vi "UPRcontroller_v00_basedonlsmv66.vi"() -> ()   [LabVIEW 2015] (continued)
                                n2048 = call "2pparameters.vi"("Params in"=w5216, "command"="set") -> ()  [unwired: 1 out]
                                }
                                frame #1 {
                                n2049 = call "waveformparamsv2.vi"("command"="rem DO", "index"=w5227) -> ()  [unwired: 3 in, 3 out]
                                }
                                frame #2 {
                                n2050 = call "waveformsDObuffer.vi"("command"="get") -> ("DO wf out"=w5233:digitalwaveform[])  [unwired: 1 in]
                                n2051 = Delete From Array(array=w5233, length=1, index=w5232) -> (array with subset deleted=w5229:digitalwaveform[])  [unwired: 1 out]
                                n2052 = call "waveformsDObuffer.vi"("DO wf in"=w5229, "command"="set") -> ()  [unwired: 1 out]
                                }
                                }
                                }
                                frame 2 {
                                n2053 = stacked-sequence {
                                tunnel: w5236 -> [_ _ w5249]
                                tunnel: w5235 -> [_ w5247 _]
                                frame #0 {
                                n2054 = call "configuration.vi"("command"="get") -> ("config out"=w5238:T14)  [unwired: 2 in, 1 out]
                                n2055 = Unbundle By Name(w5238) -> ("LT timestamp"=w5237:u32)
                                n2056 = call "2pparameters.vi"("command"="get") -> ("params out"=w5242:T12)  [unwired: 1 in]
                                n2057 = in-place {
                                in-place-border: w5237 -> [w5246]
                                n2058 = in-place-cluster #42(w5242) -> ("aDO"=w5245:u32[])
                                n2059 = call "add channel to active arrayv2.vi"("line array in"=w5245, "line to add"=w5246) -> ("line array out"=w5244:u32[])  [unwired: 2 out]
                                n2060 = in-place-cluster #42("aDO"=w5244) -> (w5240:T12)
                                }
                                n2061 = call "2pparameters.vi"("Params in"=w5240, "command"="set") -> ()  [unwired: 1 out]
                                }
                                frame #1 {
                                n2062 = call "waveformparamsv2.vi"("command"="add DO", "add DO"=w5247) -> ()  [unwired: 3 in, 3 out]
                                }
                                frame #2 {
                                n2063 = call "waveformsDObuffer.vi"("command"="get") -> ("DO wf out"=w5252:digitalwaveform[])  [unwired: 1 in]
                                n2064 = Build Array (concatenate)(w5252, w5249) -> (w5251:digitalwaveform[])
                                n2065 = call "waveformsDObuffer.vi"("DO wf in"=w5251, "command"="set") -> ()  [unwired: 1 out]
                                }
                                }
                                }
                                frame 0 {
                                n2066 = stacked-sequence {
                                seq-local: [w5258 _ _] -> [_ w5268 w5285]
                                tunnel: w5257 -> [_ _ _]
                                tunnel: w5256 -> [_ _ _]
                                tunnel: w5255 -> [_ w5265 _]
                                tunnel: w5254 -> [_ _ w5284]
                                frame #0 {
                                n2067 = call "configuration.vi"("command"="get") -> ("config out"=w5263:T14)  [unwired: 2 in, 1 out]
                                n2068 = Unbundle By Name(w5263) -> ("LT timestamp"=w5259:u32)
                                n2069 = call "2pparameters.vi"("command"="get") -> ("params out"=w5262:T12)  [unwired: 1 in]
                                n2070 = Unbundle By Name(w5262) -> ("aDO"=w5260:u32[])
                                n2071 = Search 1D Array(1D array=w5260, element=w5259) -> (index of element=w5258:i32)  [unwired: 1 in]
                                }
                                frame #1 {
                                n2072 = local read "Measurement"() -> (w5267:T4)
                                n2073 = To Unsigned Long Integer(number=w5267) -> (unsigned 32bit integer=w5266:u32)
                                n2074 = case shown="5..7" w5266 {
                                tunnel: w5268 -> [_ w5272]
                                tunnel: w5265 -> [_ w5269]
                                frame 0..4, Default {
                                }
                                frame 5..7 {
                                n2075 = Index Array(array=w5269, index=0) -> (element=w5270:T21)
                                n2076 = call "waveformparamsv2.vi"("command"="get") -> ("Params out"=w5275:T17)  [unwired: 4 in, 2 out]
                                n2077 = in-place {
                                in-place-border: w5272 -> [w5279]
                                in-place-border: w5270 -> [w5277]
                                n2078 = in-place-cluster #43(w5275) -> ("DO parameters"=w5280:T20)
                                n2079 = in-place {
                                in-place-border: w5277 -> [w5281]
                                n2080 = in-place-array #44(w5280, w5279) -> ()  [unwired: 1 out]
                                n2081 = in-place-array #44(w5281) -> (w5278:T20)  [unwired: 1 out]
                                }
                                n2082 = in-place-cluster #43("DO parameters"=w5278) -> (w5273:T17)
                                }
                                n2083 = call "waveformparamsv2.vi"("command"="set", "Params in"=w5273) -> ()  [unwired: 3 in, 3 out]
                                }
                                }
                                }
                                frame #2 {
                                n2084 = local read "Measurement"() -> (w5283:T4)
                                n2085 = To Unsigned Long Integer(number=w5283) -> (unsigned 32bit integer=w5282:u32)
                                n2086 = case shown="5..7" w5282 {
                                tunnel: w5285 -> [_ w5289]
                                tunnel: w5284 -> [_ w5287]
                                frame 0..4, Default {
                                }
                                frame 5..7 {
                                n2087 = Index Array(array=w5287, index=0) -> (element=w5286:digitalwaveform)
                                n2088 = call "waveformsDObuffer.vi"("command"="get") -> ("DO wf out"=w5291:digitalwaveform[])  [unwired: 1 in]
                                n2089 = Replace Array Subset(array=w5291, new element=w5286, index=w5289) -> (w5293:digitalwaveform[])
                                n2090 = call "waveformsDObuffer.vi"("DO wf in"=w5293, "command"="set") -> ()  [unwired: 1 out]
                                }
                                }
                                }
                                }
                                }
                                }
                              }
                              frame #4 {
                                n2091 = call "Used AO lines.vi"() -> ("used AO names"=w5296:string[], "used AO lines"=w5294:tag[])  [unwired: 2 in]
                                n2092 = control-ref of="Analog Lines Plot"() -> (w5295:refnum<vi>)
                                n2093 = control-ref of="Digital Lines Plot"() -> (w5297:refnum<vi>)
                                n2094 = call "Used DO lines.vi"() -> ("used DO names"=w5298:string[], "used DO lines"=w5299:tag[])  [unwired: 2 in]
                                n2095 = local write "Analog Used Lines"(w5294) -> ()
                                n2096 = local write "Analog Used Names"(w5296) -> ()
                                n2097 = local write "Digital Used Lines"(w5299) -> ()
                                n2098 = local write "Digital Used Names"(w5298) -> ()
                                n2099 = call "prepDOWaveplot.vi"("DigitalGraph in"=w5297, "used DO names"=w5298) -> ()  [unwired: 1 in]
                                n2100 = call "prepAOWaveplot.vi"("WaveformGraph in"=w5295, "Analog Used Names"=w5296) -> ()  [unwired: 1 in]
                              }
                              frame #5 {
                                # "source of crashing?"
                                n2101 = local read "Meastab"() -> (w5314:enum32{"X-Y Image", "Linescan", "Timetrace"})
                                n2102 = property on="refwf" class="Ring (strict)"() -> ("RingText.Text"=w5311:string)  [unwired: 2 in, 2 out]
                                n2103 = case shown="\"Timetrace\"" w5314 {
                                tunnel: [w5316 w5317] -> w5315
                                frame "X-Y Image", Default {
                                n2104 = local read "Sampling rate"() -> (w5316:dbl)
                                }
                                frame "Timetrace" {
                                n2105 = local read "srateAODOtt"() -> (w5317:dbl)
                                }
                                }
                                n2106 = call "waveformsAObuffer.vi"("command"="get") -> ("AO wf out"=w5302:waveform(dbl)[])  [unwired: 1 in]
                                n2107 = local read "wavdet"() -> (w5312:bool)
                                n2108 = call "waveformsDObuffer.vi"("command"="get") -> ("DO wf out"=w5306:digitalwaveform[])  [unwired: 1 in]
                                n2109 = call "correctwaveformsizetemp.vi"("new sampling frequency (Hz)"=w5315, "start"=FALSE, "reference waveforms to"=w5311, "Analog waveforms in"=w5302, "stop"=TRUE, "Digital waveforms in"=w5306) -> ("analog wf out"=w5308:waveform(dbl)[], "Digital wf out"=w5310:digitalwaveform[], "measpoints"=w5313:i32)
                                n2110 = local write "Analog Lines Plot"(w5308) -> ()
                                n2111 = call "GetNumCamFramesv2.vi"("Digital Waveform Graph"=w5310) -> ("Numeric"=w5309:i32)  [unwired: 10 in]
                                n2112 = local write "Digital Lines Plot"(w5310) -> ()
                                n2113 = call "waveformsDObuffer.vi"("DO wf in"=w5310, "command"="set") -> ()  [unwired: 1 out]
                                n2114 = call "waveformsAObuffer.vi"("AO wf in"=w5308, "command"="set") -> ()  [unwired: 1 out]
                                n2115 = local write "Total Camera Frames"(w5309) -> ()
                                n2116 = case shown="True" w5312 {
                                tunnel: w5313 -> [_ w5318]
                                frame False {
                                }
                                frame True {
                                n2117 = local write "# of frames"(w5318) -> ()
                                }
                                }
                              }
                            }
                          }
                          frame #9 {
                            w5328 = FALSE ("Value (Signaling)")
                            # "Save parameters, reset system..."
                            n2118 = local read "save\ndata"() -> (w5323:bool)
                            n2119 = case shown="True" w5323 {
                              tunnel: w5322 -> [_ w5335]
                              frame False {
                              }
                              frame True {
                                n2120 = call "closebinaryfiles.vi"() -> ()  [unwired: 12 in]
                                n2121 = local read "filename prefix"() -> (w5336:string)
                                n2122 = local read "data dir"() -> (w5337:path)
                                n2123 = disable-structure shown="Disabled" {
                                disable-tunnel: w5336 -> [w5340 _]
                                disable-tunnel: w5337 -> [w5339 _]
                                disable-tunnel: w5335 -> [w5338 _]
                                frame Disabled {
                                n2124 = call "saveparams.vi"("timestamp"=w5338, "filename prefix in"=w5340, "data dir in"=w5339) -> ()  [unwired: 1 in]
                                }
                                frame Enabled {
                                }
                                }
                                n2125 = call "saveparams_andscanpattern.vi"("timestamp"=w5335, "filename prefix in"=w5336, "data dir in"=w5337) -> ()  [unwired: 1 in]
                              }
                            }
                            n2126 = call "2pparameters.vi"("command"="get") -> ("params out"=w5319:T12)  [unwired: 1 in]
                            n2127 = Unbundle By Name(w5319) -> ("auto OD"=w5320:bool)
                            n2128 = case shown="True" w5320 {
                              frame False {
                              }
                              frame True {
                                n2129 = call "configuration.vi"("command"="get") -> ("config out"=w5331:T14)  [unwired: 2 in, 1 out]
                                n2130 = call "2pparameters.vi"("command"="get") -> ("params out"=w5334:T12)  [unwired: 1 in]
                                n2131 = Unbundle By Name(w5331) -> ("contour OD"=w5329:u16)
                                n2132 = Unbundle By Name(w5334) -> ("ODfilt"=w5330:u16)
                                n2133 = call "filterwheelcontrol_nothorlabslib.vi"("Current OD filt"=w5329, "New ODfilt"=w5330) -> ()  [unwired: 1 in]
                              }
                            }
                            n2134 = property on="Start" class="Bool (strict)"("Val(Sgnl)"=w5328) -> ()  [unwired: 2 in, 2 out]
                            n2135 = property on="Start" class="Bool (strict)"("Visible"=TRUE, "DisabledEnum"=T8."Enabled" ("Disabled")) -> ()  [unwired: 2 in, 2 out]
                            n2136 = property on="Stop" class="Bool (strict)"("Val(Sgnl)"=w5328) -> ()  [unwired: 2 in, 2 out]
                            n2137 = property on="Stop" class="Bool (strict)"("Visible"=FALSE, "DisabledEnum"=T8."Disabled" ("Disabled")) -> ()  [unwired: 2 in, 2 out]
                          }
                          frame #10 {
                            w5343 = T24 2 items=["no dialog", "OK message", "continue or stop message", "OK message + warnings", "continue/stop + warnings"] ("type of dialog (OK msg:1)")
                            # "Error Handling"
                            n2138 = call "displayerrors.vi"() -> ("error IO"=w5344:errorcluster)
                            n2139 = call <vilib>:"General Error Handler.vi"("type of dialog (OK msg:1)"=w5343, "error in (no error)"=w5344) -> ("error out"=w5342:errorcluster)  [unwired: 9 in, 4 out]
                            n2140 = call <vilib>:"Clear Errors.vi"("error in (no error)"=w5342) -> ("error out"=w5341:errorcluster)  [unwired: 5 in, 1 out]
                            n2141 = call "seterrors.vi"("error IO"=w5341) -> ()
                          }
                        }
                      }
                    }
                  }
                  frame "Lifetime (point)" {
                    # "Not really used"
                    # "Disabled for conversion to 64 bit"
                    n2142 = disable-structure shown="Disabled" {
                      frame Disabled {
                        n2143 = stacked-sequence {
                          frame #0 {
                            w5356 = 12.5 ("x")
                            # "get from syncrate"
                            n2144 = local read "Bin size"() -> (w5350:T7)
                            n2145 = local read "Vx-ref"() -> (w5362:dbl)
                            n2146 = local read "Vy-ref"() -> (w5363:dbl)
                            n2147 = call "2pparameters.vi"("command"="get") -> ("params out"=w5348:T12)  [unwired: 1 in]
                            n2148 = Scale By Power Of 2(n=w5350, x=1.0 ("Y Scale.Range:Minimum")) -> (x*2^n=w5359:dbl)
                            n2149 = call "setposition.vi"("Vy"=w5363, "Vx"=w5362) -> ()  [unwired: 1 in]
                            n2150 = Unbundle By Name(w5348) -> ("autoshutter"=w5349:bool, "aAS"=w5346:u32[])
                            n2151 = Multiply(x=3000.0 ("Y Scale.Range:Minimum"), y=w5359) -> (x*y=w5357:dbl)
                            n2152 = Compound Arithmetic op=MULTIPLY(w5356, invert 3200.0 ("X Scale.Offset and Multiplier:Multiplier"), w5359) -> (w5358:dbl)
                            n2153 = case shown="True" w5349 {
                              tunnel: w5346 -> [_ w5375]
                              frame False {
                              }
                              frame True {
                                n2154 = call "shuttercontrol_multi.vi"("Autoshutter Chans"=w5375, "command"="open") -> ()  [unwired: 1 in, 1 out]
                              }
                            }
                            n2155 = call "lifetimeparameters.vi"("command"="get") -> ("Params out"=w5354:T22)  [unwired: 1 in]
                            n2156 = property on="Histogram" class="WFGraph (strict)"("XScale.Maximum"=w5356, "XScale.Minimum"=0.0 ("X Scale.Range:Minimum"), "YScale.Maximum"=w5357, "YScale.Minimum"=0.1 ("Y Scale.Range:Minimum"), "XScale.Multiplier"=w5358) -> ()  [unwired: 2 in, 2 out]
                            n2157 = Bundle By Name(cluster=w5354, "Bin size"=w5350) -> (w5355:T22)
                            n2158 = call "lifetimeparameters.vi"("Params in"=w5355, "command"="set") -> ()  [unwired: 1 out]
                            n2159 = property on="Histogram 2" class="WFGraph (strict)"("YScale.Maximum"=w5357, "XScale.Multiplier"=w5358, "XScale.Maximum"=w5356) -> ()  [unwired: 2 in, 2 out]
                            n2160 = call "2pparameters.vi"("command"="get") -> ("params out"=w5370:T12)  [unwired: 1 in]
                            n2161 = Bundle By Name(cluster=w5370, "type"="Lifetime (point)") -> (w5368:T12)
                            n2162 = property on="Stop" class="Bool (strict)"("Visible"=TRUE, "DisabledEnum"=T8."Enabled" ("Disabled")) -> ()  [unwired: 2 in, 2 out]
                            n2163 = property on="Start" class="Bool (strict)"("Visible"=FALSE, "DisabledEnum"=T8."Disabled and Grayed Out" ("Disabled")) -> ()  [unwired: 2 in, 2 out]
                            n2164 = call "2pparameters.vi"("Params in"=w5368, "command"="set") -> ()  [unwired: 1 out]
                          }
                          frame #1 {
                            n2165 = call "setup.vi"() -> ()  [unwired: 1 in]
                          }
                          frame #2 {
                            # "main loop"
                            n2166 = call "lifetimeparameters.vi"("command"="get") -> ("Params out"=w5381:T22)  [unwired: 1 in]
                            n2167 = Unbundle By Name(w5381) -> ("devidx"=w5379:i32)
                            n2168 = for {
                              N: 10000 -> [_]
                              tunnel: [w5382] -> w5377 mode=indexing
                              i -> [w5382]
                            }
                            n2169 = while {
                              tunnel: w5379 -> [w5386]
                              tunnel: w5377 -> [w5383]
                              i -> [w5384]
                              stop <- w5388 stop-if-true
                              n2170 = Increment(x=w5384) -> (x+1=w5385:i32)
                              n2171 = dll-call lib="phlib.dll" fn="_PH_GetCountRate@8" label="PH_GetCountRate"("devidx"=w5386, "channel"=0) -> (w5387:i32)  [unwired: 5 in, 2 out]
                              "SyncRate" <- w5387
                              n2172 = stacked-sequence {
                                seq-local: [_ _ w5395 _ _] -> [_ _ _ w5408 _]
                                seq-local: [_ _ w5394 _ _] -> [_ _ _ w5407 _]
                                seq-local: [_ w5392 _ _ _] -> [_ _ w5396 _ _]
                                tunnel: w5387 -> [_ _ _ w5415 _]
                                tunnel: w5383 -> [_ _ _ w5405 _]
                                frame #0 {
                                n2173 = call "start_binned.vi"() -> ()  [unwired: 1 in]
                                }
                                frame #1 {
                                n2174 = call "get-histogram.vi"() -> ("IntegralCount"=→"Integral count":u32, "Histogram"=w5392:u32[])
                                "Histogram" <- w5392
                                }
                                frame #2 {
                                n2175 = Search 1D Array(1D array=w5396, element=u32 0) -> (index of element=w5394:i32)  [unwired: 1 in]
                                n2176 = Multiply(x=w5394, y=0.99) -> (x*y=w5400:dbl)
                                n2177 = Array Subset(array=w5396, index=0, length=w5400) -> (w5403:u32[])
                                n2178 = Array Max & Min(array=w5403) -> (max index (indices)=w5397:i32)  [unwired: 3 out]
                                n2179 = Split 1D Array(array=w5403, index=w5397) -> (second subarray=w5399:u32[])  [unwired: 1 out]
                                n2180 = Array Max & Min(array=w5399) -> (min index (indices)=w5398:i32)  [unwired: 3 out]
                                n2181 = Split 1D Array(array=w5399, index=w5398) -> (first subarray=w5395:u32[])  [unwired: 1 out]
                                "Histogram 2" <- w5395
                                }
                                frame #3 {
                                n2182 = Array Size(array=w5408) -> (size(s)=w5410:i32)
                                n2183 = Array Subset(array=w5405, index=0, length=w5410) -> (w5409:i32[])
                                n2184 = Compound Arithmetic op=MULTIPLY(1000000000.0 ("value"), invert w5415, invert w5407, w5409) -> (w5406:dbl[])
                                n2185 = call <vilib>:"Exponential Fit.vi"("Y"=w5408, "X"=w5406) -> ("damping"=w5412:dbl)  [unwired: 8 in, 5 out]
                                n2186 = Divide(x=-1.0 ("y"), y=w5412) -> (x/y=→"Lifetime (ns)":dbl)
                                }
                                frame #4 {
                                n2187 = local read "downright"() -> (w5422:bool)
                                n2188 = local read "downleft"() -> (w5424:bool)
                                n2189 = local read "upright"() -> (w5420:bool)
                                n2190 = local read "upleft"() -> (w5418:bool)
                                n2191 = local read "down"() -> (w5423:bool)
                                n2192 = local read "right"() -> (w5421:bool)
                                n2193 = local read "left"() -> (w5425:bool)
                                n2194 = local read "up"() -> (w5419:bool)
                                n2195 = Compound Arithmetic op=OR(w5418, w5419, w5420, w5421, w5422, w5423, w5424, w5425) -> (w5417:bool)
                                n2196 = case shown="True" w5417 {
                                frame False {
                                }
                                frame True {
                                n2197 = stacked-sequence {
                                frame #0 {
                                n2198 = local read "downright"() -> (w5427:bool)
                                n2199 = local read "downleft"() -> (w5429:bool)
                                n2200 = local read "BigSmall"() -> (w5426:bool)
                                n2201 = local read "upright"() -> (w5431:bool)
                                n2202 = local read "upleft"() -> (w5434:bool)
                                n2203 = local read "down"() -> (w5430:bool)
                                n2204 = local read "right"() -> (w5432:bool)
                                n2205 = local read "left"() -> (w5428:bool)
                                n2206 = local read "up"() -> (w5433:bool)
                                n2207 = call "movestageparams.vi"("command"="get") -> ("Params out"=w5437:T23)  [unwired: 1 in]
                                n2208 = Bundle By Name(cluster=w5437, "upleft"=w5434, "up"=w5433, "upright"=w5431, "right"=w5432, "downright"=w5427, "down"=w5430, "downleft"=w5429, "left"=w5428, "Bigsmall"=w5426) -> (w5438:T23)
                                n2209 = call "movestageparams.vi"("Params in"=w5438, "command"="set") -> ()  [unwired: 1 out]
                                }
                                frame #1 {
                                n2210 = call "movestage.vi"() -> ()  [unwired: 12 in]
                                }
                                frame #2 {
                                w5439 = FALSE ("OK Button")
                                w5440 = FALSE ("OK Button")
                                n2211 = property on="down" class="Bool (strict)"("Value"=w5440) -> ()  [unwired: 2 in, 2 out]
                                n2212 = property on="up" class="Bool (strict)"("Value"=w5440) -> ()  [unwired: 2 in, 2 out]
                                n2213 = property on="right" class="Bool (strict)"("Value"=w5440) -> ()  [unwired: 2 in, 2 out]
                                n2214 = property on="left" class="Bool (strict)"("Value"=w5440) -> ()  [unwired: 2 in, 2 out]
                                n2215 = property on="upleft" class="Bool (strict)"("Value"=w5439) -> ()  [unwired: 2 in, 2 out]
                                n2216 = property on="upright" class="Bool (strict)"("Value"=w5439) -> ()  [unwired: 2 in, 2 out]
                                n2217 = property on="downleft" class="Bool (strict)"("Value"=w5439) -> ()  [unwired: 2 in, 2 out]
                                n2218 = property on="downright" class="Bool (strict)"("Value"=w5439) -> ()  [unwired: 2 in, 2 out]
                                }
                                }
                                }
                                }
                                }
                              }
                              n2219 = dll-call lib="phlib.dll" fn="_PH_GetCountRate@8" label="PH_GetCountRate"("devidx"=w5386, "channel"=1) -> (→"Ch1Rate":i32)  [unwired: 5 in, 2 out]
                              n2220 = local read "Stop"() -> (w5388:bool)
                              n2221 = local write "points recorded"(w5385) -> ()
                            }
                          }
                          frame #3 {
                            w5449 = FALSE ("Value (Signaling)")
                            n2222 = call "2pparameters.vi"("command"="get") -> ("params out"=w5443:T12)  [unwired: 1 in]
                            n2223 = Unbundle By Name(w5443) -> ("autoshutter"=w5444:bool, "aAS"=w5441:u32[])
                            n2224 = case shown="True" w5444 {
                              tunnel: w5441 -> [_ w5450]
                              frame False {
                              }
                              frame True {
                                n2225 = call "shuttercontrol_multi.vi"("Autoshutter Chans"=w5450, "command"="close") -> ()  [unwired: 1 in, 1 out]
                              }
                            }
                            n2226 = property on="Start" class="Bool (strict)"("Val(Sgnl)"=w5449) -> ()  [unwired: 2 in, 2 out]
                            n2227 = property on="Start" class="Bool (strict)"("Visible"=TRUE, "DisabledEnum"=T8."Enabled" ("Disabled")) -> ()  [unwired: 2 in, 2 out]
                            n2228 = property on="Stop" class="Bool (strict)"("Val(Sgnl)"=w5449) -> ()  [unwired: 2 in, 2 out]
                            n2229 = property on="Stop" class="Bool (strict)"("Visible"=FALSE, "DisabledEnum"=T8."Disabled" ("Disabled")) -> ()  [unwired: 2 in, 2 out]
                          }
                        }
                      }
                      frame Enabled {
                      }
                    }
                    n2230 = local write "64bit disabled"(TRUE ("64bit disabled")) -> ()
                  }
                }
              }
            }
          }
          event "avpp", "Angle ref", "xpixels ref", "Vx-min ref", "Vx-max ref", "ypixels ref", "Vy-min ref", "Vy-max ref", "ROI Type", "Sampling rate": Value Change {
            n2231 = event-data() -> ()  [unwired: 1 in, 6 out]
            n2232 = local read "avpp"() -> (w5469:i32)
            n2233 = local read "Angle ref"() -> (w5468:dbl)
            n2234 = local read "ROI Type"() -> (w5467:u16)
            n2235 = local read "xpixels ref"() -> (w5464:i32)
            n2236 = local read "Vx-min ref"() -> (w5463:dbl)
            n2237 = local read "Vx-max ref"() -> (w5462:dbl)
            n2238 = local read "ypixels ref"() -> (w5460:i32)
            n2239 = local read "Vy-min ref"() -> (w5461:dbl)
            n2240 = local read "Vy-max ref"() -> (w5457:dbl)
            n2241 = local read "Sampling rate"() -> (w5452:dbl)
            n2242 = local read "# of frames"() -> (w5456:i32)
            n2243 = local read "maxbufferAI"() -> (w5455:i32)
            n2244 = local read "Override AI buffer"() -> (w5453:bool)
            n2245 = call "2pparameters.vi"("command"="get") -> ("params out"=w5466:T12)  [unwired: 1 in]
            n2246 = Bundle By Name(cluster=w5466, "avpp"=w5469, "Angle Img"=w5468, "Xpixels Img"=w5464, "Vx-min Img"=w5463, "VX-max Img"=w5462, "Ypixels Img"=w5460, "Vy-min Img"=w5461, "Vy-max Img"=w5457, "srate"=w5452, "srate Img"=w5452, "measpoints"=w5456, "maxbufferAI"=w5455, "Drawing Mode"=w5467, "Vz-reset"=0.0, "AIoverride"=w5453) -> (w5458:T12)
            n2247 = call "2pparameters.vi"("Params in"=w5458, "command"="set") -> ()  [unwired: 1 out]
          }
          event "# of frames": Value Change {
            n2248 = event-data() -> ()  [unwired: 1 in, 6 out]
            n2249 = local read "Meastab"() -> (w5470:enum32{"X-Y Image", "Linescan", "Timetrace"})
            n2250 = case shown="\"Linescan\"" w5470 {
              frame "X-Y Image", Default {
                n2251 = local read "# of frames"() -> (w5471:i32)
                n2252 = call "2pparameters.vi"("command"="get") -> ("params out"=w5475:T12)  [unwired: 1 in]
                n2253 = Bundle By Name(cluster=w5475, "measpoints"=w5471) -> (w5472:T12)
                n2254 = call "2pparameters.vi"("Params in"=w5472, "command"="set") -> ()  [unwired: 1 out]
              }
              frame "Linescan" {
                n2255 = local read "srateAODOtt"() -> (w5485:dbl)
                n2256 = local read "# of frames"() -> (w5481:i32)
                n2257 = local read "refreshtime"() -> (w5487:dbl)
                n2258 = local read "bin"() -> (w5482:dbl)
                n2259 = call "tt_timeandsamples.vi"("bin"=w5482, "refreshtime"=w5487, "srateAODOtt"=w5485, "tot#ofsamples"=w5481) -> ("refreshrate"=w5484:dbl, "refreshbuffer"=w5483:i32, "timetracecycles"=w5480:i32)  [unwired: 5 in]
                n2260 = call "2pparameters.vi"("command"="get") -> ("params out"=w5477:T12)  [unwired: 1 in]
                n2261 = Bundle By Name(cluster=w5477, "measpoints"=w5481, "tt_cycles"=w5480, "refreshbuffer"=w5483, "refreshrate"=w5484) -> (w5479:T12)
                n2262 = Reciprocal(x=w5484) -> (1/x=w5486:dbl)
                n2263 = local write "refreshtime"(w5486) -> ()
                n2264 = call "2pparameters.vi"("Params in"=w5479, "command"="set") -> ()  [unwired: 1 out]
              }
              frame "Timetrace" {
                n2265 = local read "srateAODOtt"() -> (w5497:dbl)
                n2266 = local read "# of frames"() -> (w5493:i32)
                n2267 = local read "refreshtime"() -> (w5499:dbl)
                n2268 = local read "bin"() -> (w5494:dbl)
                n2269 = call "tt_timeandsamples.vi"("bin"=w5494, "refreshtime"=w5499, "srateAODOtt"=w5497, "tot#ofsamples"=w5493) -> ("refreshrate"=w5496:dbl, "refreshbuffer"=w5495:i32, "timetracecycles"=w5492:i32)  [unwired: 5 in]
                n2270 = call "2pparameters.vi"("command"="get") -> ("params out"=w5489:T12)  [unwired: 1 in]
                n2271 = Bundle By Name(cluster=w5489, "measpoints"=w5493, "tt_cycles"=w5492, "refreshbuffer"=w5495, "refreshrate"=w5496) -> (w5491:T12)
                n2272 = Reciprocal(x=w5496) -> (1/x=w5498:dbl)
                n2273 = local write "refreshtime"(w5498) -> ()
                n2274 = call "2pparameters.vi"("Params in"=w5491, "command"="set") -> ()  [unwired: 1 out]
              }
            }
          }
          event "srateAODOtt", "refreshtime", "Vx-ref", "Vy-ref", "Vx-min draw", "Vx-max draw", "Vy-min draw", "Vy-max draw", "bin": Value Change {
            n2275 = event-data() -> ()  [unwired: 1 in, 6 out]
            n2276 = local read "ypixels ref"() -> (w5531:i32)
            n2277 = local read "Vy-min draw"() -> (w5507:dbl)
            n2278 = local read "Vy-max draw"() -> (w5506:dbl)
            n2279 = local read "Vx-min draw"() -> (w5509:dbl)
            n2280 = local read "Vx-max draw"() -> (w5508:dbl)
            n2281 = local read "xpixels ref"() -> (w5505:i32)
            n2282 = local read "ROI Type"() -> (w5504:u16)
            n2283 = local read "Pel"() -> (w5503:dbl)
            n2284 = local read "srateAODOtt"() -> (w5513:dbl)
            n2285 = local read "# of frames"() -> (w5518:i32)
            n2286 = local read "refreshtime"() -> (w5511:dbl)
            n2287 = local read "bin"() -> (w5516:dbl)
            n2288 = local read "Override AI buffer"() -> (w5501:bool)
            n2289 = local read "finite samples"() -> (w5525:bool)
            n2290 = local read "srateAODOtt"() -> (w5500:dbl)
            n2291 = local read "srateAODOtt"() -> (w5519:dbl)
            n2292 = local read "continuous"() -> (w5524:bool)
            n2293 = local read "Angle ref"() -> (w5510:dbl)
            n2294 = local read "wavdet"() -> (w5526:bool)
            n2295 = local read "Vx-ref"() -> (w5521:dbl)
            n2296 = local read "Vy-ref"() -> (w5523:dbl)
            n2297 = local read "avpp"() -> (w5522:i32)
            n2298 = call "tt_timeandsamples.vi"("bin"=w5516, "refreshtime"=w5511, "srateAODOtt"=w5513, "tot#ofsamples"=w5518) -> ("refreshrate"=w5514:dbl, "refreshbuffer"=w5515:i32, "timetracecycles"=w5520:i32)  [unwired: 5 in]
            n2299 = local read "bin"() -> (w5517:dbl)
            n2300 = call "2pparameters.vi"("command"="get") -> ("params out"=w5529:T12)  [unwired: 1 in]
            n2301 = Bundle By Name(cluster=w5529, "Drawing Mode"=w5504, "measpoints"=w5518, "tt_cycles"=w5520, "refreshbuffer"=w5515, "refreshrate"=w5514, "Vx-ref"=w5521, "Vy-ref"=w5523, "srate"=w5500, "finite"=w5525, "cont"=w5524, "wavdet"=w5526, "avpp"=w5522, "srateAODO"=w5519, "bufferAI"=w5515, "bin"=w5517, "Angle Img"=w5510, "Vxminref"=w5509, "Vxmaxref"=w5508, "Vyminref"=w5507, "Vymaxref"=w5506, "Xpixels Img"=w5505, "Ypixels Img"=w5531, "Pel"=w5503, "Vz-reset"=0.0, "AIoverride"=w5501) -> (w5527:T12)
            n2302 = Reciprocal(x=w5514) -> (1/x=w5512:dbl)
            n2303 = local write "refreshtime"(w5512) -> ()
            n2304 = call "2pparameters.vi"("Params in"=w5527, "command"="set") -> ()  [unwired: 1 out]
          }
          event "Init": Value Change {
            # "Disabled for conversion to 64 bit"
            n2305 = event-data() -> ()  [unwired: 1 in, 6 out]
            n2306 = disable-structure shown="Disabled" {
              frame Disabled {
                n2307 = flat-sequence {
                  frame #0 {
                    n2308 = local read "Measurement"() -> (w5533:T4)
                    n2309 = case shown="\"Lifetime (scan)\", \"Lifetime (contour)\"" w5533 {
                      frame "X-Y-t movie", Default {
                      }
                      frame "Lifetime (point)" {
                        n2310 = stacked-sequence {
                          frame #0 {
                            n2311 = call "initialize.vi"("mode"=0) -> ()
                          }
                          frame #1 {
                            n2312 = call "calib.vi"() -> ()  [unwired: 1 in]
                          }
                        }
                      }
                      frame "Lifetime (scan)", "Lifetime (contour)" {
                        n2313 = stacked-sequence {
                          frame #0 {
                            n2314 = call "initialize.vi"("mode"=3) -> ()
                          }
                          frame #1 {
                            n2315 = call "calib.vi"() -> ()  [unwired: 1 in]
                          }
                        }
                      }
                    }
                  }
                  frame #1 {
                    n2316 = property on="Start" class="Bool (strict)"("Visible"=TRUE, "DisabledEnum"=T8."Enabled" ("Disabled")) -> ()  [unwired: 2 in, 2 out]
                    n2317 = property on="Init" class="Bool (strict)"("Visible"=FALSE, "DisabledEnum"=T8."Disabled and Grayed Out" ("Disabled"), "Value"=FALSE ("Init")) -> ()  [unwired: 2 in, 2 out]
                  }
                }
              }
              frame Enabled {
              }
            }
            n2318 = local write "64bit disabled"(TRUE ("64bit disabled")) -> ()
          }
          event "Measurement": Value Change {
            n2319 = event-data() -> ()  [unwired: 1 in, 5 out]
            n2320 = case shown="\"X-Y-Z stack\"" "Measurement" {
              frame "X-Y-t movie" {
                w5548 = T8."Disabled" ("Disabled")
                w5547 = FALSE ("Visible")
                n2321 = call "2pparameters.vi"("command"="get") -> ("params out"=w5558:T12)  [unwired: 1 in]
                n2322 = local write "graphtab"(T5."image" ("graphtab")) -> ()
                n2323 = local write "Save tab"(enum32{"withsave", "withoutsave"}."withsave" ("Save tab")) -> ()
                n2324 = Bundle By Name(cluster=w5558, "type"="X-Y-t movie") -> (w5556:T12)
                n2325 = call "2pparameters.vi"("Params in"=w5556, "command"="set") -> ()  [unwired: 1 out]
                n2326 = property on="refreshtime" class="DigNum (strict)"("Visible"=FALSE, "DisabledEnum"=T8."Disabled and Grayed Out" ("Disabled")) -> ()  [unwired: 2 in, 2 out]
                n2327 = property on="Start" class="Bool (strict)"("Visible"=TRUE, "DisabledEnum"=T8."Enabled" ("Disabled")) -> ()  [unwired: 2 in, 2 out]
                n2328 = property on="Init" class="Bool (strict)"("Visible"=FALSE, "DisabledEnum"=T8."Disabled and Grayed Out" ("Disabled"), "Value"=FALSE ("Init")) -> ()  [unwired: 2 in, 2 out]
                n2329 = property on="ttt" class="Enum (strict)"("Visible"=FALSE) -> ()  [unwired: 2 in, 2 out]
                n2330 = property on="# of frames" class="DigNum (strict)"("DisabledEnum"=T8."Enabled" ("Disabled"), "Caption.Text"="# of frames") -> ()  [unwired: 2 in, 2 out]
                n2331 = property on="continuous" class="Bool (strict)"("Visible"=TRUE, "DisabledEnum"=T8."Enabled" ("Disabled")) -> ()  [unwired: 2 in, 2 out]
                n2332 = property on="finite samples" class="Bool (strict)"("Visible"=TRUE, "DisabledEnum"=T8."Enabled" ("Disabled")) -> ()  [unwired: 2 in, 2 out]
                n2333 = property on="avpp" class="DigNum (strict)"("Visible"=TRUE, "DisabledEnum"=T8."Enabled" ("Disabled")) -> ()  [unwired: 2 in, 2 out]
                n2334 = property on="srateAODOtt" class="DigNum (strict)"("Visible"=FALSE, "DisabledEnum"=T8."Disabled" ("Disabled")) -> ()  [unwired: 2 in, 2 out]
                n2335 = local write "save\ndata"(TRUE ("save\ndata")) -> ()
                n2336 = property on="finite samples" class="Bool (strict)"("Val(Sgnl)"=TRUE ("continuous for display")) -> ()  [unwired: 2 in, 2 out]
                n2337 = property on="continuous" class="Bool (strict)"("Value"=FALSE ("continuous for display")) -> ()  [unwired: 2 in, 2 out]
                n2338 = property on="Current Average" class="DigNum (strict)"("Visible"=TRUE, "DisabledEnum"=T8."Enabled" ("Disabled")) -> ()  [unwired: 2 in, 2 out]
                n2339 = property on="img_CH1" class="IntGraph (strict)"("ZScale.Maximum"=7.0 ("Z Scale.Range:Maximum")) -> ()  [unwired: 2 in, 2 out]
                n2340 = property on="Sampling rate" class="DigNum (strict)"("Visible"=TRUE, "DisabledEnum"=T8."Enabled" ("Disabled")) -> ()  [unwired: 2 in, 2 out]
                n2341 = property on="Pel" class="DigNum (strict)"("Visible"=w5547, "DisabledEnum"=w5548) -> ()  [unwired: 2 in, 2 out]
                n2342 = property on="bin" class="DigNum (strict)"("Visible"=w5547, "DisabledEnum"=w5548) -> ()  [unwired: 2 in, 2 out]
                "Meastab" <- enum32{"X-Y Image", "Linescan", "Timetrace"}."X-Y Image" ("Meastab")
                "Zscantab" <- enum32{"withzscan", "withoutzscan", "lifetime"}."withoutzscan" ("Zscantab")
              }
              frame "X-Y-Z stack" {
                w5585 = T8."Disabled" ("Disabled")
                w5584 = FALSE ("Visible")
                n2343 = call "2pparameters.vi"("command"="get") -> ("params out"=w5595:T12)  [unwired: 1 in]
                n2344 = call "2pparameters.vi"("command"="get") -> ("params out"=w5599:T12)  [unwired: 1 in]
                n2345 = Bundle By Name(cluster=w5595, "type"="X-Y-Z stack") -> (w5593:T12)
                n2346 = Unbundle By Name(w5599) -> ("motorref"=w5598:refnum<k7>)
                n2347 = call "2pparameters.vi"("Params in"=w5593, "command"="set") -> ()  [unwired: 1 out]
                n2348 = local write "Zscantab"(enum32{"withzscan", "withoutzscan", "lifetime"}."withzscan" ("Zscantab")) -> ()
                n2349 = local write "Meastab"(enum32{"X-Y Image", "Linescan", "Timetrace"}."X-Y Image" ("Meastab")) -> ()
                n2350 = invoke class="MG17Motor" method="GetPosition"(reference=w5598, "lChanID"=0, "pfPosition"=sgl 0.0) -> ("pfPosition"=w5610:sgl)  [unwired: 2 in, 4 out]
                n2351 = property on="refreshtime" class="DigNum (strict)"("Visible"=FALSE, "DisabledEnum"=T8."Disabled and Grayed Out" ("Disabled")) -> ()  [unwired: 2 in, 2 out]
                n2352 = property on="Start" class="Bool (strict)"("Visible"=TRUE, "DisabledEnum"=T8."Enabled" ("Disabled")) -> ()  [unwired: 2 in, 2 out]
                n2353 = property on="Init" class="Bool (strict)"("Visible"=FALSE, "DisabledEnum"=T8."Disabled and Grayed Out" ("Disabled"), "Value"=FALSE ("Init")) -> ()  [unwired: 2 in, 2 out]
                n2354 = property on="ttt" class="Enum (strict)"("Visible"=FALSE) -> ()  [unwired: 2 in, 2 out]
                n2355 = Multiply(x=w5610, y=1000.0) -> (x*y=w5609:dbl)
                n2356 = local write "Actual Z position"(w5609) -> ()
                n2357 = local write "Save tab"(enum32{"withsave", "withoutsave"}."withsave" ("Save tab")) -> ()
                n2358 = property on="finite samples" class="Bool (strict)"("Visible"=FALSE, "DisabledEnum"=T8."Disabled and Grayed Out" ("Disabled")) -> ()  [unwired: 2 in, 2 out]
                n2359 = property on="avpp" class="DigNum (strict)"("Visible"=TRUE, "DisabledEnum"=T8."Enabled" ("Disabled")) -> ()  [unwired: 2 in, 2 out]
                n2360 = property on="continuous" class="Bool (strict)"("Visible"=FALSE, "DisabledEnum"=T8."Disabled and Grayed Out" ("Disabled")) -> ()  [unwired: 2 in, 2 out]
                n2361 = property on="img_CH1" class="IntGraph (strict)"("ZScale.Maximum"=7.0 ("Z Scale.Range:Maximum")) -> ()  [unwired: 2 in, 2 out]
                n2362 = property on="srateAODOtt" class="DigNum (strict)"("Visible"=FALSE, "DisabledEnum"=T8."Disabled" ("Disabled")) -> ()  [unwired: 2 in, 2 out]
                n2363 = property on="Pel" class="DigNum (strict)"("Visible"=w5584, "DisabledEnum"=w5585) -> ()  [unwired: 2 in, 2 out]
                n2364 = property on="bin" class="DigNum (strict)"("Visible"=w5584, "DisabledEnum"=w5585) -> ()  [unwired: 2 in, 2 out]
                n2365 = property on="Current Average" class="DigNum (strict)"("Visible"=TRUE, "DisabledEnum"=T8."Enabled" ("Disabled")) -> ()  [unwired: 2 in, 2 out]
                n2366 = property on="# of frames" class="DigNum (strict)"("Caption.Text"="# of slices", "DisabledEnum"=T8."Disabled and Grayed Out" ("Disabled")) -> ()  [unwired: 2 in, 2 out]
                n2367 = local write "save\ndata"(TRUE ("save\ndata")) -> ()
                n2368 = property on="finite samples" class="Bool (strict)"("Val(Sgnl)"=TRUE ("continuous for display")) -> ()  [unwired: 2 in, 2 out]
                n2369 = property on="continuous" class="Bool (strict)"("Value"=FALSE ("continuous for display")) -> ()  [unwired: 2 in, 2 out]
                n2370 = property on="Sampling rate" class="DigNum (strict)"("Visible"=TRUE, "DisabledEnum"=T8."Enabled" ("Disabled")) -> ()  [unwired: 2 in, 2 out]
              }
              frame "X-Y-Z-t movie" {
                w5629 = T8."Disabled" ("Disabled")
                w5628 = FALSE ("Visible")
                n2371 = property on="# of frames" class="DigNum (strict)"("DisabledEnum"=T8."Enabled" ("Disabled")) -> ()  [unwired: 2 in, 2 out]
                n2372 = property on="Current Average" class="DigNum (strict)"("Visible"=TRUE, "DisabledEnum"=T8."Enabled" ("Disabled")) -> ()  [unwired: 2 in, 2 out]
                n2373 = property on="avpp" class="DigNum (strict)"("Visible"=TRUE, "DisabledEnum"=T8."Enabled" ("Disabled")) -> ()  [unwired: 2 in, 2 out]
                n2374 = local write "Save tab"(enum32{"withsave", "withoutsave"}."withsave" ("Save tab")) -> ()
                n2375 = local write "Zscantab"(enum32{"withzscan", "withoutzscan", "lifetime"}."withzscan" ("Zscantab")) -> ()
                n2376 = local write "Meastab"(enum32{"X-Y Image", "Linescan", "Timetrace"}."X-Y Image" ("Meastab")) -> ()
                n2377 = property on="Start" class="Bool (strict)"("Visible"=TRUE, "DisabledEnum"=T8."Enabled" ("Disabled")) -> ()  [unwired: 2 in, 2 out]
                n2378 = property on="refreshtime" class="DigNum (strict)"("Visible"=FALSE, "DisabledEnum"=T8."Disabled and Grayed Out" ("Disabled")) -> ()  [unwired: 2 in, 2 out]
                n2379 = property on="Init" class="Bool (strict)"("Visible"=FALSE, "DisabledEnum"=T8."Disabled and Grayed Out" ("Disabled"), "Value"=FALSE ("Init")) -> ()  [unwired: 2 in, 2 out]
                n2380 = property on="ttt" class="Enum (strict)"("Visible"=FALSE) -> ()  [unwired: 2 in, 2 out]
                n2381 = call "2pparameters.vi"("command"="get") -> ("params out"=w5639:T12)  [unwired: 1 in]
                n2382 = Bundle By Name(cluster=w5639, "type"="X-Y-Z-t movie") -> (w5637:T12)
                n2383 = property on="continuous" class="Bool (strict)"("Visible"=TRUE, "DisabledEnum"=T8."Enabled" ("Disabled")) -> ()  [unwired: 2 in, 2 out]
                n2384 = property on="finite samples" class="Bool (strict)"("Visible"=TRUE, "DisabledEnum"=T8."Enabled" ("Disabled")) -> ()  [unwired: 2 in, 2 out]
                n2385 = call "2pparameters.vi"("Params in"=w5637, "command"="set") -> ()  [unwired: 1 out]
                n2386 = property on="srateAODOtt" class="DigNum (strict)"("Visible"=FALSE, "DisabledEnum"=T8."Disabled" ("Disabled")) -> ()  [unwired: 2 in, 2 out]
                n2387 = local write "save\ndata"(TRUE ("save\ndata")) -> ()
                n2388 = property on="img_CH1" class="IntGraph (strict)"("ZScale.Maximum"=7.0 ("Z Scale.Range:Maximum")) -> ()  [unwired: 2 in, 2 out]
                n2389 = property on="continuous" class="Bool (strict)"("Value"=FALSE ("continuous for display")) -> ()  [unwired: 2 in, 2 out]
                n2390 = property on="finite samples" class="Bool (strict)"("Value"=TRUE ("continuous for display")) -> ()  [unwired: 2 in, 2 out]
                n2391 = property on="Sampling rate" class="DigNum (strict)"("Visible"=TRUE, "DisabledEnum"=T8."Enabled" ("Disabled")) -> ()  [unwired: 2 in, 2 out]
                n2392 = property on="Pel" class="DigNum (strict)"("Visible"=w5628, "DisabledEnum"=w5629) -> ()  [unwired: 2 in, 2 out]
                n2393 = property on="bin" class="DigNum (strict)"("Visible"=w5628, "DisabledEnum"=w5629) -> ()  [unwired: 2 in, 2 out]
              }
              frame "linescan" {
                w5664 = T8."Enabled" ("Disabled")
                w5663 = TRUE ("Visible")
                w5666 = T8."Enabled" ("Disabled")
                w5665 = TRUE ("Visible")
                n2394 = local write "Meastab"(enum32{"X-Y Image", "Linescan", "Timetrace"}."Linescan" ("Meastab")) -> ()
                n2395 = property on="Current Average" class="DigNum (strict)"("Visible"=TRUE, "DisabledEnum"=T8."Enabled" ("Disabled")) -> ()  [unwired: 2 in, 2 out]
                n2396 = property on="ttt" class="Enum (strict)"("Visible"=FALSE) -> ()  [unwired: 2 in, 2 out]
                n2397 = local write "Save tab"(enum32{"withsave", "withoutsave"}."withsave" ("Save tab")) -> ()
                n2398 = local write "Zscantab"(enum32{"withzscan", "withoutzscan", "lifetime"}."withoutzscan" ("Zscantab")) -> ()
                n2399 = property on="refreshtime" class="DigNum (strict)"("Visible"=FALSE, "DisabledEnum"=T8."Disabled and Grayed Out" ("Disabled")) -> ()  [unwired: 2 in, 2 out]
                n2400 = property on="continuous" class="Bool (strict)"("Value"=FALSE ("continuous for display")) -> ()  [unwired: 2 in, 2 out]
                n2401 = property on="finite samples" class="Bool (strict)"("Value"=TRUE ("continuous for display")) -> ()  [unwired: 2 in, 2 out]
                n2402 = local write "save\ndata"(TRUE ("save\ndata")) -> ()
                n2403 = property on="Start" class="Bool (strict)"("Visible"=TRUE, "DisabledEnum"=T8."Enabled" ("Disabled")) -> ()  [unwired: 2 in, 2 out]
                n2404 = property on="Init" class="Bool (strict)"("Visible"=FALSE, "DisabledEnum"=T8."Disabled and Grayed Out" ("Disabled"), "Value"=FALSE ("Init")) -> ()  [unwired: 2 in, 2 out]
                n2405 = call "2pparameters.vi"("command"="get") -> ("params out"=w5675:T12)  [unwired: 1 in]
                n2406 = Bundle By Name(cluster=w5675, "type"="linescan") -> (w5673:T12)
                n2407 = property on="# of frames" class="DigNum (strict)"("DisabledEnum"=T8."Enabled" ("Disabled"), "Caption.Text"="# of lines") -> ()  [unwired: 2 in, 2 out]
                n2408 = property on="continuous" class="Bool (strict)"("Visible"=TRUE, "DisabledEnum"=T8."Enabled" ("Disabled")) -> ()  [unwired: 2 in, 2 out]
                n2409 = property on="avpp" class="DigNum (strict)"("Visible"=TRUE, "DisabledEnum"=T8."Enabled" ("Disabled")) -> ()  [unwired: 2 in, 2 out]
                n2410 = property on="finite samples" class="Bool (strict)"("Visible"=TRUE, "DisabledEnum"=T8."Enabled" ("Disabled")) -> ()  [unwired: 2 in, 2 out]
                n2411 = property on="srateAODOtt" class="DigNum (strict)"("Visible"=TRUE, "DisabledEnum"=T8."Enabled" ("Disabled")) -> ()  [unwired: 2 in, 2 out]
                n2412 = call "2pparameters.vi"("Params in"=w5673, "command"="set") -> ()  [unwired: 1 out]
                n2413 = property on="Pel" class="DigNum (strict)"("Visible"=w5665, "DisabledEnum"=w5666) -> ()  [unwired: 2 in, 2 out]
                n2414 = property on="bin" class="DigNum (strict)"("Visible"=w5665, "DisabledEnum"=w5666) -> ()  [unwired: 2 in, 2 out]
                n2415 = property on="Sampling rate" class="DigNum (strict)"("Visible"=FALSE, "DisabledEnum"=T8."Disabled" ("Disabled")) -> ()  [unwired: 2 in, 2 out]
                n2416 = property on="Pel" class="DigNum (strict)"("Visible"=w5663, "DisabledEnum"=w5664) -> ()  [unwired: 2 in, 2 out]
                n2417 = property on="bin" class="DigNum (strict)"("Visible"=w5663, "DisabledEnum"=w5664) -> ()  [unwired: 2 in, 2 out]
              }
              frame "Timetrace" {
                w5701 = T8."Enabled" ("Disabled")
                w5700 = TRUE ("Visible")
                n2418 = call "2pparameters.vi"("command"="get") -> ("params out"=w5706:T12)  [unwired: 1 in]
                n2419 = local write "Meastab"(enum32{"X-Y Image", "Linescan", "Timetrace"}."Timetrace" ("Meastab")) -> ()
                n2420 = Unbundle By Name(w5706) -> ("Angle draw"=w5708:dbl)
                n2421 = local write "Zscantab"(enum32{"withzscan", "withoutzscan", "lifetime"}."withoutzscan" ("Zscantab")) -> ()
                n2422 = property on="# of frames" class="DigNum (strict)"("DisabledEnum"=T8."Enabled" ("Disabled"), "Caption.Text"="# of samples") -> ()  [unwired: 2 in, 2 out]
                n2423 = property on="refreshtime" class="DigNum (strict)"("Visible"=TRUE, "DisabledEnum"=T8."Enabled" ("Disabled")) -> ()  [unwired: 2 in, 2 out]
                n2424 = property on="avpp" class="DigNum (strict)"("Visible"=FALSE, "DisabledEnum"=T8."Disabled and Grayed Out" ("Disabled")) -> ()  [unwired: 2 in, 2 out]
                n2425 = property on="Current Average" class="DigNum (strict)"("Visible"=FALSE, "DisabledEnum"=T8."Disabled and Grayed Out" ("Disabled")) -> ()  [unwired: 2 in, 2 out]
                n2426 = local write "Angle drawing"(w5708) -> ()
                n2427 = property on="ttt" class="Enum (strict)"("Visible"=TRUE) -> ()  [unwired: 2 in, 2 out]
                n2428 = property on="continuous" class="Bool (strict)"("Visible"=TRUE, "DisabledEnum"=T8."Enabled" ("Disabled")) -> ()  [unwired: 2 in, 2 out]
                n2429 = property on="finite samples" class="Bool (strict)"("Visible"=TRUE, "DisabledEnum"=T8."Enabled" ("Disabled")) -> ()  [unwired: 2 in, 2 out]
                n2430 = local write "save\ndata"(TRUE ("save\ndata")) -> ()
                n2431 = property on="finite samples" class="Bool (strict)"("Val(Sgnl)"=TRUE ("continuous for display")) -> ()  [unwired: 2 in, 2 out]
                n2432 = property on="continuous" class="Bool (strict)"("Value"=FALSE ("continuous for display")) -> ()  [unwired: 2 in, 2 out]
                n2433 = local write "Save tab"(enum32{"withsave", "withoutsave"}."withsave" ("Save tab")) -> ()
                n2434 = property on="srateAODOtt" class="DigNum (strict)"("Visible"=TRUE, "DisabledEnum"=T8."Enabled" ("Disabled")) -> ()  [unwired: 2 in, 2 out]
                n2435 = call "2pparameters.vi"("command"="get") -> ("params out"=w5713:T12)  [unwired: 1 in]
                n2436 = property on="Start" class="Bool (strict)"("Visible"=TRUE, "DisabledEnum"=T8."Enabled" ("Disabled")) -> ()  [unwired: 2 in, 2 out]
                n2437 = property on="Init" class="Bool (strict)"("Visible"=FALSE, "DisabledEnum"=T8."Disabled and Grayed Out" ("Disabled"), "Value"=FALSE ("Init")) -> ()  [unwired: 2 in, 2 out]
                n2438 = Bundle By Name(cluster=w5713, "type"="Timetrace") -> (w5711:T12)
                n2439 = property on="Sampling rate" class="DigNum (strict)"("Visible"=FALSE, "DisabledEnum"=T8."Disabled" ("Disabled")) -> ()  [unwired: 2 in, 2 out]
                n2440 = property on="Pel" class="DigNum (strict)"("Visible"=w5700, "DisabledEnum"=w5701) -> ()  [unwired: 2 in, 2 out]
                n2441 = property on="bin" class="DigNum (strict)"("Visible"=w5700, "DisabledEnum"=w5701) -> ()  [unwired: 2 in, 2 out]
                n2442 = call "2pparameters.vi"("Params in"=w5711, "command"="set") -> ()  [unwired: 1 out]
              }
              frame "Lifetime (point)" {
                w5734 = T8."Enabled" ("Disabled")
                w5733 = TRUE ("Visible")
                n2443 = property on="Pel" class="DigNum (strict)"("Visible"=w5733, "DisabledEnum"=w5734) -> ()  [unwired: 2 in, 2 out]
                n2444 = property on="bin" class="DigNum (strict)"("Visible"=w5733, "DisabledEnum"=w5734) -> ()  [unwired: 2 in, 2 out]
                n2445 = property on="ttt" class="Enum (strict)"("Visible"=FALSE) -> ()  [unwired: 2 in, 2 out]
                n2446 = local write "Zscantab"(enum32{"withzscan", "withoutzscan", "lifetime"}."lifetime" ("Zscantab")) -> ()
                n2447 = local write "graphtab"(T5."Lifetime" ("graphtab")) -> ()
                n2448 = local write "Meastab"(enum32{"X-Y Image", "Linescan", "Timetrace"}."Timetrace" ("Meastab")) -> ()
                n2449 = call "lifetimeparameters.vi"("command"="get") -> ("Params out"=w5741:T22)  [unwired: 1 in]
                n2450 = Unbundle By Name(w5741) -> ("initialized"=w5742:bool)
                n2451 = property on="srateAODOtt" class="DigNum (strict)"("Visible"=TRUE, "DisabledEnum"=T8."Enabled" ("Disabled")) -> ()  [unwired: 2 in, 2 out]
                n2452 = case shown="False" w5742 {
                  frame False {
                    n2453 = property on="Init" class="Bool (strict)"("Visible"=TRUE, "DisabledEnum"=T8."Enabled" ("Disabled")) -> ()  [unwired: 2 in, 2 out]
                    n2454 = property on="Start" class="Bool (strict)"("Visible"=FALSE, "DisabledEnum"=T8."Disabled and Grayed Out" ("Disabled")) -> ()  [unwired: 2 in, 2 out]
                  }
                  frame True {
                  }
                }
                n2455 = property on="Sampling rate" class="DigNum (strict)"("Visible"=FALSE, "DisabledEnum"=T8."Disabled" ("Disabled")) -> ()  [unwired: 2 in, 2 out]
              }
              frame "Lifetime (scan)" {
                w5751 = T8."Disabled" ("Disabled")
                w5750 = FALSE ("Visible")
                n2456 = call "lifetimeparameters.vi"("command"="get") -> ("Params out"=w5763:T22)  [unwired: 1 in]
                n2457 = local write "graphtab"(T5."image" ("graphtab")) -> ()
                n2458 = local write "Save tab"(enum32{"withsave", "withoutsave"}."withsave" ("Save tab")) -> ()
                n2459 = local write "Meastab"(enum32{"X-Y Image", "Linescan", "Timetrace"}."X-Y Image" ("Meastab")) -> ()
                n2460 = local write "Zscantab"(enum32{"withzscan", "withoutzscan", "lifetime"}."lifetime" ("Zscantab")) -> ()
                n2461 = Unbundle By Name(w5763) -> ("initialized"=w5762:bool)
                n2462 = property on="ttt" class="Enum (strict)"("Visible"=FALSE) -> ()  [unwired: 2 in, 2 out]
                n2463 = property on="refreshtime" class="DigNum (strict)"("Visible"=FALSE, "DisabledEnum"=T8."Disabled and Grayed Out" ("Disabled")) -> ()  [unwired: 2 in, 2 out]
                n2464 = property on="Pel" class="DigNum (strict)"("Visible"=w5750, "DisabledEnum"=w5751) -> ()  [unwired: 2 in, 2 out]
                n2465 = property on="bin" class="DigNum (strict)"("Visible"=w5750, "DisabledEnum"=w5751) -> ()  [unwired: 2 in, 2 out]
                n2466 = property on="save data" class="Bool (strict)"("Visible"=TRUE, "DisabledEnum"=T8."Enabled" ("Disabled"), "Value"=TRUE ("Visible")) -> ()  [unwired: 2 in, 2 out]
                n2467 = case shown="False" w5762 {
                  frame False {
                    n2468 = property on="Init" class="Bool (strict)"("Visible"=TRUE, "DisabledEnum"=T8."Enabled" ("Disabled")) -> ()  [unwired: 2 in, 2 out]
                    n2469 = property on="Start" class="Bool (strict)"("Visible"=FALSE, "DisabledEnum"=T8."Disabled and Grayed Out" ("Disabled")) -> ()  [unwired: 2 in, 2 out]
                  }
                  frame True {
                  }
                }
                n2470 = call "2pparameters.vi"("command"="get") -> ("params out"=w5768:T12)  [unwired: 1 in]
                n2471 = property on="continuous" class="Bool (strict)"("Visible"=TRUE, "DisabledEnum"=T8."Disabled and Grayed Out" ("Disabled")) -> ()  [unwired: 2 in, 2 out]
                n2472 = property on="finite samples" class="Bool (strict)"("Visible"=TRUE, "DisabledEnum"=T8."Enabled" ("Disabled")) -> ()  [unwired: 2 in, 2 out]
                n2473 = Bundle By Name(cluster=w5768, "type"="Lifetime (scan)") -> (w5766:T12)
                n2474 = call "2pparameters.vi"("Params in"=w5766, "command"="set") -> ()  [unwired: 1 out]
                n2475 = property on="finite samples" class="Bool (strict)"("Val(Sgnl)"=TRUE ("continuous for display")) -> ()  [unwired: 2 in, 2 out]
                n2476 = property on="continuous" class="Bool (strict)"("Value"=FALSE ("continuous for display")) -> ()  [unwired: 2 in, 2 out]
                n2477 = property on="srateAODOtt" class="DigNum (strict)"("Visible"=FALSE, "DisabledEnum"=T8."Disabled" ("Disabled")) -> ()  [unwired: 2 in, 2 out]
                n2478 = property on="# of frames" class="DigNum (strict)"("DisabledEnum"=T8."Enabled" ("Disabled"), "Caption.Text"="# of frames") -> ()  [unwired: 2 in, 2 out]
                n2479 = property on="img_CH1" class="IntGraph (strict)"("ZScale.Maximum"=12.5 ("Z Scale.Range:Maximum")) -> ()  [unwired: 2 in, 2 out]
                n2480 = property on="Current Average" class="DigNum (strict)"("Visible"=TRUE, "DisabledEnum"=T8."Enabled" ("Disabled")) -> ()  [unwired: 2 in, 2 out]
                n2481 = property on="Sampling rate" class="DigNum (strict)"("Visible"=TRUE, "DisabledEnum"=T8."Enabled" ("Disabled")) -> ()  [unwired: 2 in, 2 out]
                n2482 = property on="avpp" class="DigNum (strict)"("Visible"=TRUE, "DisabledEnum"=T8."Enabled" ("Disabled")) -> ()  [unwired: 2 in, 2 out]
              }
              frame "Lifetime (contour)" {
                w5792 = T8."Enabled" ("Disabled")
                w5791 = TRUE ("Visible")
                n2483 = call "2pparameters.vi"("command"="get") -> ("params out"=w5799:T12)  [unwired: 1 in]
                n2484 = property on="# of frames" class="DigNum (strict)"("DisabledEnum"=T8."Enabled" ("Disabled"), "Caption.Text"="# of samples") -> ()  [unwired: 2 in, 2 out]
                n2485 = property on="refreshtime" class="DigNum (strict)"("Visible"=TRUE, "DisabledEnum"=T8."Enabled" ("Disabled")) -> ()  [unwired: 2 in, 2 out]
                n2486 = Unbundle By Name(w5799) -> ("Angle draw"=w5801:dbl)
                n2487 = property on="avpp" class="DigNum (strict)"("Visible"=FALSE, "DisabledEnum"=T8."Disabled and Grayed Out" ("Disabled")) -> ()  [unwired: 2 in, 2 out]
                n2488 = property on="Current Average" class="DigNum (strict)"("Visible"=FALSE, "DisabledEnum"=T8."Disabled and Grayed Out" ("Disabled")) -> ()  [unwired: 2 in, 2 out]
                n2489 = local write "Angle drawing"(w5801) -> ()
                n2490 = local write "Save tab"(enum32{"withsave", "withoutsave"}."withsave" ("Save tab")) -> ()
                n2491 = local write "Zscantab"(enum32{"withzscan", "withoutzscan", "lifetime"}."lifetime" ("Zscantab")) -> ()
                n2492 = local write "graphtab"(T5."Lifetime" ("graphtab")) -> ()
                n2493 = local write "Meastab"(enum32{"X-Y Image", "Linescan", "Timetrace"}."Timetrace" ("Meastab")) -> ()
                n2494 = property on="ttt" class="Enum (strict)"("Visible"=TRUE) -> ()  [unwired: 2 in, 2 out]
                n2495 = call "lifetimeparameters.vi"("command"="get") -> ("Params out"=w5823:T22)  [unwired: 1 in]
                n2496 = property on="finite samples" class="Bool (strict)"("Val(Sgnl)"=TRUE ("continuous for display")) -> ()  [unwired: 2 in, 2 out]
                n2497 = local write "save\ndata"(TRUE ("save\ndata")) -> ()
                n2498 = Unbundle By Name(w5823) -> ("initialized"=w5824:bool)
                n2499 = property on="continuous" class="Bool (strict)"("Visible"=TRUE, "DisabledEnum"=T8."Enabled" ("Disabled")) -> ()  [unwired: 2 in, 2 out]
                n2500 = property on="finite samples" class="Bool (strict)"("Visible"=TRUE, "DisabledEnum"=T8."Enabled" ("Disabled")) -> ()  [unwired: 2 in, 2 out]
                n2501 = property on="Pel" class="DigNum (strict)"("Visible"=w5791, "DisabledEnum"=w5792) -> ()  [unwired: 2 in, 2 out]
                n2502 = property on="bin" class="DigNum (strict)"("Visible"=w5791, "DisabledEnum"=w5792) -> ()  [unwired: 2 in, 2 out]
                n2503 = property on="continuous" class="Bool (strict)"("Value"=FALSE ("continuous for display")) -> ()  [unwired: 2 in, 2 out]
                n2504 = case shown="False" w5824 {
                  frame False {
                    n2505 = property on="Init" class="Bool (strict)"("Visible"=TRUE, "DisabledEnum"=T8."Enabled" ("Disabled")) -> ()  [unwired: 2 in, 2 out]
                    n2506 = property on="Start" class="Bool (strict)"("Visible"=FALSE, "DisabledEnum"=T8."Disabled and Grayed Out" ("Disabled")) -> ()  [unwired: 2 in, 2 out]
                  }
                  frame True {
                  }
                }
